vi "benchmarks_largeBinarySHA1.vi"() -> ()   [LabVIEW 2013]
uses:
  SHA-1/SHA-1.lvclass
  <vilib>/Analysis/baseanly.llb/Mean (DBL).vi
  <vilib>/Analysis/NI_AALBase.lvlib
  SHA-1/SHA-1.lvlib
panel:
  out "equal hashes":bool
  out "% gain":dbl
  out "LVOS":dbl
  out "NI Forums":dbl
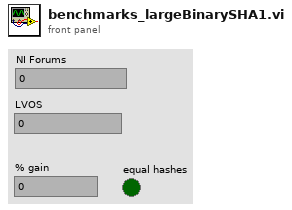
[diagram p1: front panel]
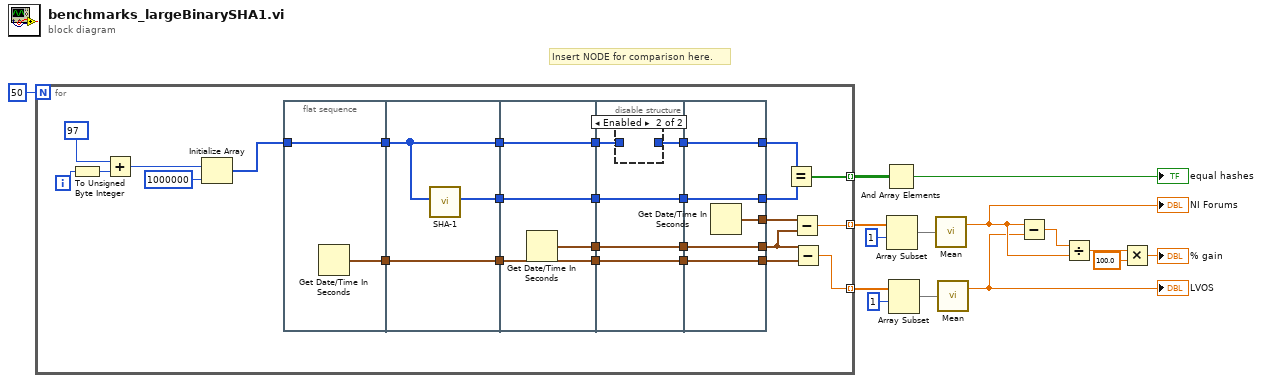
[diagram p0: block diagram]
diagram:
  # "Insert NODE for comparison here."
  n1 = for {
    N: 50 -> [_]
    tunnel: [w27] -> w15 mode=indexing
    tunnel: [w26] -> w8 mode=indexing
    tunnel: [w25] -> w7 mode=indexing
    i -> [w19]
    n2 = To Unsigned Byte Integer(number=w19) -> (unsigned 8bit integer=w16:u8)
    n3 = Add(x=u8 97 ("Numeric"), y=w16) -> (x+y=w17:u8)
    n4 = Initialize Array(w17, 1000000 ("dimension size")) -> (w20:u8[])
    n5 = flat-sequence {
      tunnel: w20 -> [w44]
      tunnel: [w44] -> w42
      tunnel: [w43] -> w41
      tunnel: [w46] -> w40
      tunnel: w42 -> [w46]
      tunnel: w41 -> [w47]
      tunnel: [w47] -> w39
      tunnel: [w45] -> w24
      tunnel: w40 -> [w51]
      tunnel: [w51] -> w38
      tunnel: [w50] -> w37
      tunnel: [w49] -> w36
      tunnel: w39 -> [w49]
      tunnel: w24 -> [w48]
      tunnel: [w48] -> w23
      tunnel: w38 -> [w53]
      tunnel: [w56] -> w35
      tunnel: w37 -> [w56]
      tunnel: [w55] -> w34
      tunnel: w36 -> [w55]
      tunnel: [w52] -> w33
      tunnel: w23 -> [w54]
      tunnel: [w54] -> w22
      tunnel: [w62] -> w31
      tunnel: w35 -> [w62]
      tunnel: [w61] -> w30
      tunnel: w34 -> [w61]
      tunnel: [w60] -> w32
      tunnel: [w59] -> w29
      tunnel: w33 -> [w59]
      tunnel: [w58] -> w28
      tunnel: w22 -> [w58]
      frame #0 {
        n6 = Get Date/Time In Seconds() -> (seconds since 1Jan1904=w43:timestamp)
      }
      frame #1 {
        n7 = call "SHA-1.vi"("data"=w46) -> ("SHA-1 hash"=w45:u8[])  [unwired: 10 in]
      }
      frame #2 {
        n8 = Get Date/Time In Seconds() -> (seconds since 1Jan1904=w50:timestamp)
      }
      frame #3 {
        n9 = disable-structure shown="Enabled" {
          disable-tunnel: [w57 _] -> w52
          disable-tunnel: w53 -> [w57 _]
          frame Disabled {
          }
          frame Enabled {
          }
        }
      }
      frame #4 {
        n10 = Get Date/Time In Seconds() -> (seconds since 1Jan1904=w60:timestamp)
      }
    }
    n11 = Equal?(x=w29, y=w28) -> (x = y?=w27:bool[])
    n12 = Subtract(x=w32, y=w31) -> (x-y=w26:dbl)
    n13 = Subtract(x=w31, y=w30) -> (x-y=w25:dbl)
  }
  n14 = And Array Elements(Boolean array=w15) -> (logical AND=→"equal hashes":bool)
  n15 = Array Subset(array=w8, index=1) -> (w11:dbl[])  [unwired: 1 in]
  n16 = Array Subset(array=w7, index=1) -> (w10:dbl[])  [unwired: 1 in]
  n17 = call-poly <vilib>:"Mean.vi"("X"=w11) -> ("mean"=w3:dbl)  [unwired: 1 out]
  "NI Forums" <- w3
  n18 = call-poly <vilib>:"Mean.vi"("X"=w10) -> ("mean"=w2:dbl)  [unwired: 1 out]
  "LVOS" <- w2
  n19 = Subtract(x=w3, y=w2) -> (x-y=w6:dbl)
  n20 = Divide(x=w6, y=w3) -> (x/y=w4:dbl)
  n21 = Multiply(x=w4, y=100.0) -> (x*y=→"% gain":dbl)
